vi "Extract Number.vi"(11 "input string":string) -> (3 "Array":i32[](array[numeric]))   [LabVIEW 2023]
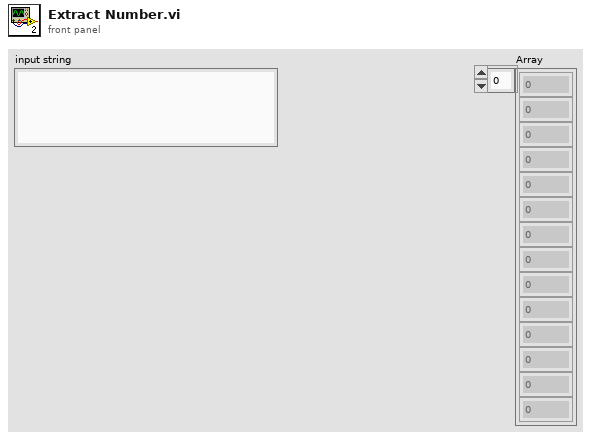
[diagram p1: front panel]
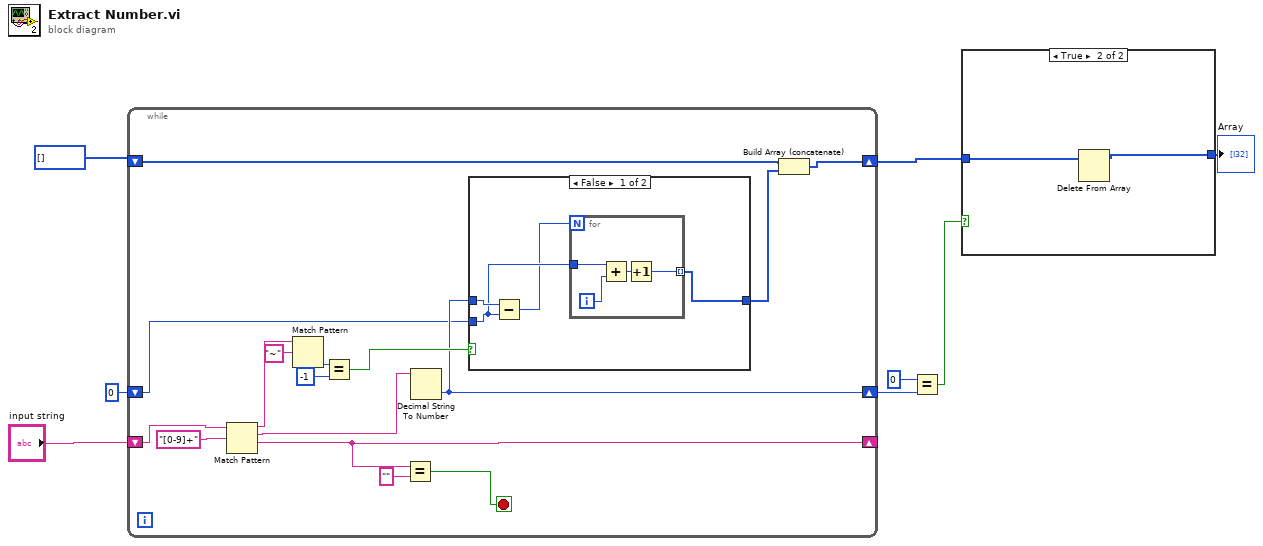
[diagram p0: block diagram]
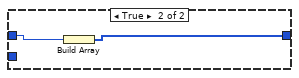
[diagram p3: hidden frame]
diagram:
  n1 = while {
    shift-right: [w21] -> _
    shift-left: "input string" -> [w20]
    shift-right: [w14] -> w5
    shift-left: 0 -> [w11]
    shift-right: [w10] -> w2
    shift-left: i32[] [] -> [w12]
    stop <- w22 stop-if-true
    n2 = Match Pattern(string=w20, regular expression="[0-9]+" ("format string")) -> (before substring=w19:string, match substring=w9:string, after substring=w21:string)  [unwired: 1 in, 1 out]
    n3 = Match Pattern(string=w19, regular expression="~") -> (offset past match=w17:i32)  [unwired: 1 in, 3 out]
    n4 = Equal?(x=w17, y=-1) -> (x = y?=w15:bool)
    n5 = Equal?(x=w21, y="") -> (x = y?=w22:bool)
    n6 = Decimal String To Number(string=w9) -> (number=w14:i32)  [unwired: 2 in, 1 out]
    n7 = case shown="False" w15 {
      tunnel: w14 -> [w28 w34]
      tunnel: [w26 w33] -> w13
      tunnel: w11 -> [w27 _]
      frame False {
        n8 = Subtract(x=w28, y=w27) -> (x-y=w25:i32)
        n9 = for {
          N: w25 -> [_]
          tunnel: w27 -> [w32]
          tunnel: [w29] -> w26 mode=indexing
          i -> [w31]
          n10 = Add(x=w32, y=w31) -> (x+y=w30:i32)
          n11 = Increment(x=w30) -> (x+1=w29:i32)
        }
      }
      frame True {
        n12 = Build Array(w34) -> (w33:i32[])
      }
    }
    n13 = Build Array (concatenate)(w12, w13) -> (w10:i32[])
  }
  n14 = Equal?(x=0, y=w5) -> (x = y?=w3:bool)
  n15 = case shown="True" w3 {
    tunnel: w2 -> [w35 w37]
    tunnel: [w35 w36] -> w1
    frame False {
    }
    frame True {
      n16 = Delete From Array(array=w37) -> (array with subset deleted=w36:i32[])  [unwired: 2 in, 1 out]
    }
  }
  "Array" <- w1
